vi "Configure Output Range.vi"(8 "error in (no error)":errorcluster, 9 "Range (High Voltage / Low Current)":string(combo)="HIGH", 11 "VISA resource name":refnum<visa-resource-name>) -> (0 "error out":errorcluster, 3 "VISA resource name out":refnum<visa-resource-name>)   [LabVIEW 2013]
doc: "Configures the power supply's output range on a channel. You specify whether you want to configure the voltage and the value to which to set the range.\n\nNotes:\n\n1) Setting a voltage range can invalidate a previously configured current range.\n\n2) Setting a current range can invalidate a previously configured voltage range."
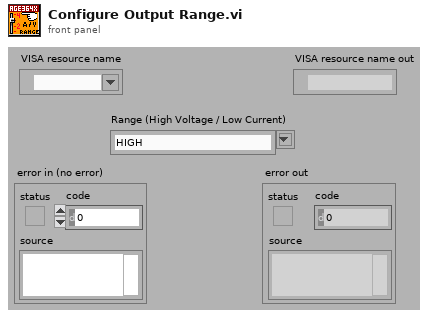
[diagram p1: front panel]
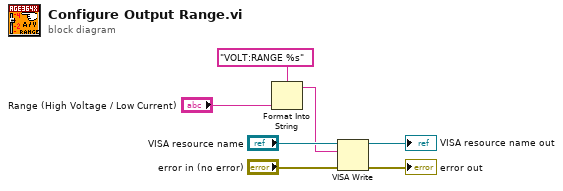
[diagram p0: block diagram]
diagram:
  n1 = Format Into String(format string="VOLT:RANGE %s", "Range (High Voltage / Low Current)") -> (resulting string=w3:string)  [unwired: 2 in, 1 out]
  n2 = VISA Write(VISA resource name="VISA resource name", write buffer=w3, error in (no error)="error in (no error)") -> (VISA resource name out=→"VISA resource name out":refnum<visa-resource-name>, error out=→"error out":errorcluster)  [unwired: 1 out]
